vi "GetDAQtiveChannelNumber.vi"(3 "error in (no error)":errorcluster, 4 "# DAQ channels":i32, 5 "Channel Settings":T1(array[cluster])) -> (0 "error out":errorcluster, 2 "# of active channels":i32)   [LabVIEW 2015]
doc: "Acquires total number of DAQtive channels per given card. To be nested within a higher-level 'for' loop in order to access other cards. The numeric output of this VI determines the # of iterations the DAQ channel storage VI will run."
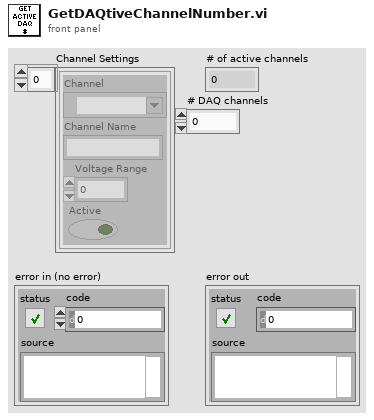
[diagram p1: front panel]
types:
  T1 = cluster{"Channel":tag, "Channel Name":string, "Voltage Range":dbl, "Active":bool}[]
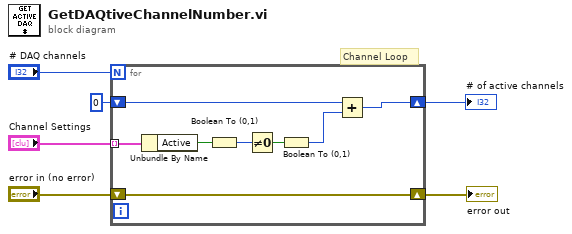
[diagram p0: block diagram]
diagram:
  # "Channel Loop"
  n1 = for {
    N: "# DAQ channels" -> [_]
    tunnel: "Channel Settings" -> [w14] mode=indexing
    shift-right: [w13] -> w3
    shift-left: "error in (no error)" -> [w13]
    shift-right: [w11] -> w6
    shift-left: 0 -> [w12]
    n2 = Unbundle By Name(w14) -> ("Active"=w9:bool)
    n3 = Boolean To (0,1)(Boolean=w9) -> (0, 1=w8:i16)
    n4 = Not Equal To 0?(x=w8) -> (x != 0?=w10:bool)
    n5 = Boolean To (0,1)(Boolean=w10) -> (0, 1=w7:i16)
    n6 = Add(x=w12, y=w7) -> (x+y=w11:i32)
  }
  "# of active channels" <- w6
  "error out" <- w3
